vi "Register Listener.vi"(8 "error in (no error)":errorcluster, 9 "Data Msg":refnum<class "Data Msg.lvclass">, 10 "Listener NQR":refnum<class "Message Enqueuer.lvclass">, 11 "Broadcast Registry In":refnum<class "Broadcast Registry.lvclass">) -> (0 "error out":errorcluster, 3 "Broadcast Registry Out":refnum<class "Broadcast Registry.lvclass">)   [LabVIEW 2016, in "Data Broadcasting.lvlib" / "Broadcast Registry.lvclass"]
doc: "Registers a Listener to receive the next broadcast of this Registry's data message. Listeners are referenced by their <b>NQR</b> (Enqueuer). When a broadcast is issued, each listener is sent its own concrete <b>Data Msg</b>.\n\n-------------\nCopyright (c) 2013, Staab Engineering, a Texas Limited Liability Company\nAll rights reserved.\n\nRedistribution and use in source and binary forms, with or without modification, are permitted provided that the following conditions are met:\n\n1. Redistributions of source code must retain the above copyright notice, this list of conditions and the following disclaimer.\n2. Redistributions in binary form must reproduce the above copyright notice, this list of conditions and the following disclaimer in the documentation and/or other materials provided with the distribution.\n\nTHIS SOFTWARE IS PROVIDED BY THE COPYRIGHT HOLDERS AND CONTRIBUTORS \"AS IS\" AND ANY EXPRESS OR IMPLIED WARRANTIES, INCLUDING, BUT NOT LIMITED TO, THE IMPLIED WARRANTIES OF MERCHANTABILITY AND FITNESS FOR A PARTICULAR PURPOSE ARE DISCLAIMED. IN NO EVENT SHALL THE COPYRIGHT HOLDER OR CONTRIBUTORS BE LIABLE FOR ANY DIRECT, INDIRECT, INCIDENTAL, SPECIAL, EXEMPLARY, OR CONSEQUENTIAL DAMAGES (INCLUDING, BUT NOT LIMITED TO, PROCUREMENT OF SUBSTITUTE GOODS OR SERVICES; LOSS OF USE, DATA, OR PROFITS; OR BUSINESS INTERRUPTION) HOWEVER CAUSED AND ON ANY THEORY OF LIABILITY, WHETHER IN CONTRACT, STRICT LIABILITY, OR TORT (INCLUDING NEGLIGENCE OR OTHERWISE) ARISING IN ANY WAY OUT OF THE USE OF THIS SOFTWARE, EVEN IF ADVISED OF THE POSSIBILITY OF SUCH DAMAGE."
uses:
  <userlib>/_Frameworks/Staab/AF Data Broadcasting/Data Broadcasting/Broadcast Registry/Broadcast Registry.lvclass
  <vilib>/ActorFramework/Message Enqueuer/Message Enqueuer.lvclass
  <userlib>/_Frameworks/Staab/AF Data Broadcasting/Data Broadcasting/Data Msg/Data Msg.lvclass
  <userlib>/_Frameworks/Staab/AF Data Broadcasting/Data Broadcasting/Broadcast Registry/Broadcast Registry.lvclass/Broadcast Registry.ctl
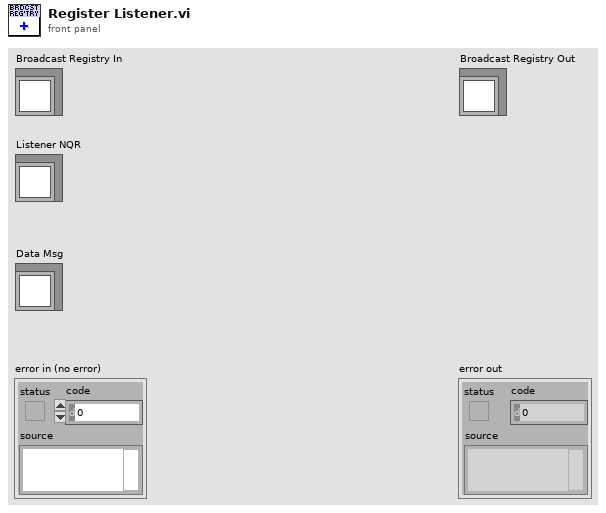
[diagram p1: front panel]
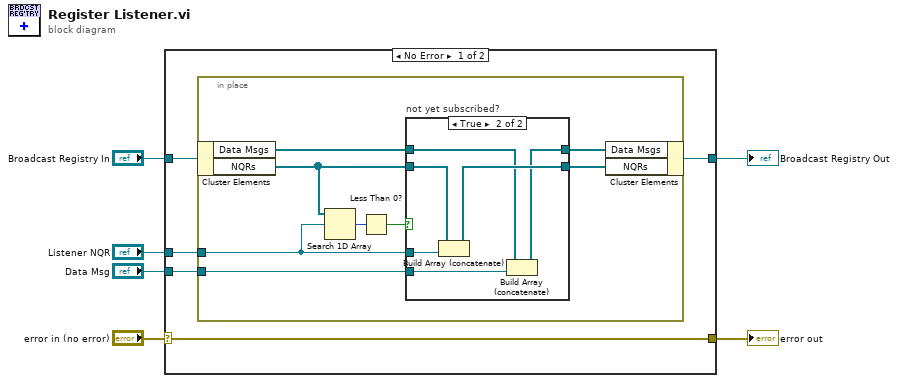
[diagram p0: block diagram]
diagram:
  n1 = case shown="No Error" "error in (no error)" {
    selector: "error in (no error)" -> [w11 w29]
    tunnel: [w11 w29] -> w5
    tunnel: [w8 w28] -> w3
    tunnel: "Broadcast Registry In" -> [w10 w28]
    tunnel: "Listener NQR" -> [w9 _]
    tunnel: "Data Msg" -> [w7 _]
    frame No Error {
      n2 = in-place {
        in-place-border: w9 -> [w15]
        in-place-border: w7 -> [w14]
        n3 = in-place-cluster #1(w10) -> ("Data Msgs"=w13:refnum<class "Data Msg.lvclass">[], "NQRs"=w16:refnum<class "Message Enqueuer.lvclass">[])
        n4 = Search 1D Array(1D array=w16, element=w15) -> (index of element=w19:i32)  [unwired: 1 in]
        n5 = Less Than 0?(x=w19) -> (x < 0?=w17:bool)
        n6 = case "not yet subscribed?" shown="True" w17 {
          tunnel: w16 -> [w21 w27]
          tunnel: [w21 w26] -> w18
          tunnel: w15 -> [_ w24]
          tunnel: w14 -> [_ w22]
          tunnel: w13 -> [w20 w25]
          tunnel: [w20 w23] -> w12
          frame False {
          }
          frame True {
            n7 = Build Array (concatenate)(w27, w24) -> (w26:refnum<class "Message Enqueuer.lvclass">[])
            n8 = Build Array (concatenate)(w25, w22) -> (w23:refnum<class "Data Msg.lvclass">[])
          }
        }
        n9 = in-place-cluster #1("Data Msgs"=w12, "NQRs"=w18) -> (w8:refnum<class "Broadcast Registry.lvclass">)
      }
    }
    frame Error {
    }
  }
  "error out" <- w5
  "Broadcast Registry Out" <- w3
